vi "Set Configuration.vi"(8 "error in (no error)":errorcluster, 10 "configuration":T1={"name"="", "components"=[], "cycle timing"={"priority"=10000, "decimation"=1, "offset"=0}}, 11 "Core Plugins Configuration in":refnum<class "Core Plugin Configuration.lvclass">) -> (0 "error out":errorcluster, 3 "Core Plugins Configuration out":refnum<class "Core Plugin Configuration.lvclass">)   [LabVIEW 2017, in "DSF Core.lvlib" / "Core Plugin Configuration.lvclass"]
uses:
  Core Plugin Configuration.lvclass
  Typedefs/DSF Core Plugin Configuration.ctl
  Typedefs/DSF Timing Info.ctl
  Core Plugin Configuration.lvclass/Core Plugin Configuration.ctl
  DSF Core.lvlib
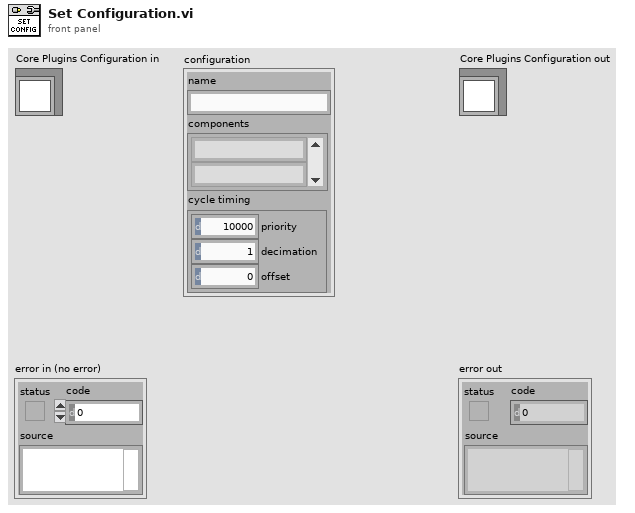
[diagram p1: front panel]
types:
  T1 = typedef "DSF Core.lvlib/DSF Core Plugin Configuration.ctl" = cluster{"name":string, "components":string[], "cycle timing":T2}
  T2 = typedef "DSF Core.lvlib/DSF Timing Info.ctl" = cluster{"priority":u64, "decimation":u64, "offset":u64}
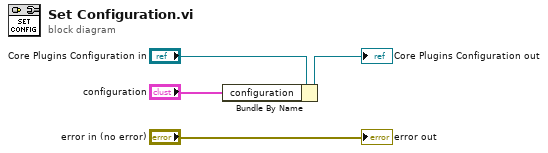
[diagram p0: block diagram]
diagram:
  n1 = Bundle By Name(cluster="Core Plugins Configuration in", "configuration"="configuration") -> (→"Core Plugins Configuration out":refnum<class "Core Plugin Configuration.lvclass">)
  "error out" <- "error in (no error)"
